vi "Run Command.vi"(8 "error in (no error)":errorcluster, 11 "Console Wrapper in":refnum<class "Console Wrapper.lvclass">) -> (0 "error out":errorcluster, 3 "Console Wrapper out":refnum<class "Console Wrapper.lvclass">)   [LabVIEW 2020, in "Console Wrapper.lvclass"]
doc: "Runs a built command in a specified working directory in the command line. It will wait until the command processing is finished and will not display the console window."
uses:
  Console Wrapper.lvclass
  Read Command.vi
  Read Working Directory.vi
  Write Standard Output.vi
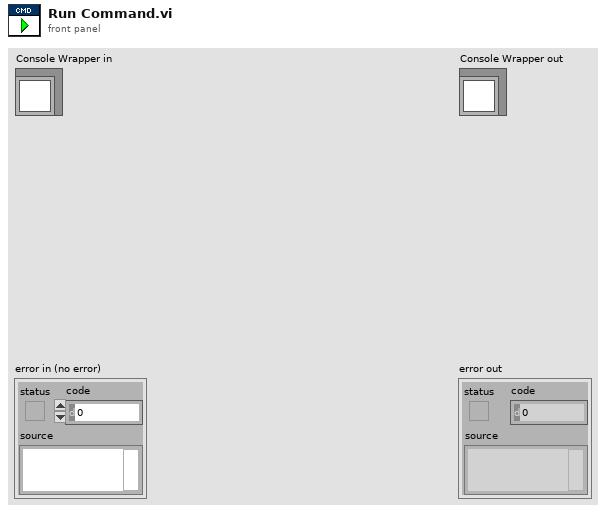
[diagram p1: front panel]
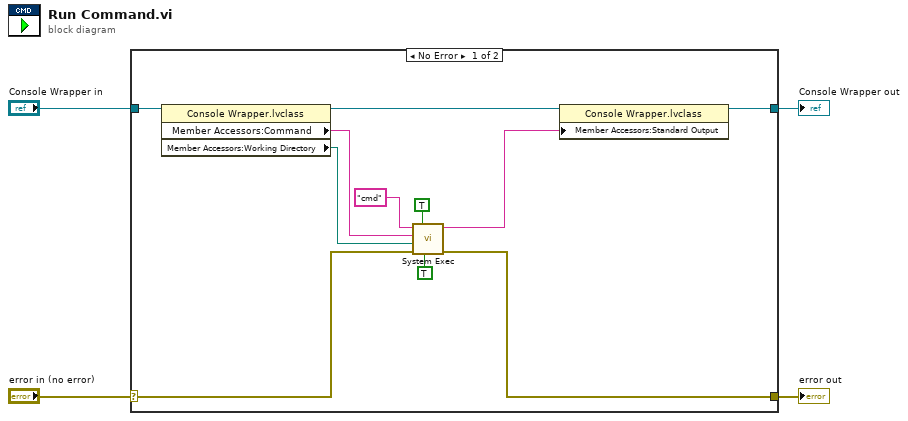
[diagram p0: block diagram]
diagram:
  n1 = case shown="No Error" "error in (no error)" {
    selector: "error in (no error)" -> [w6 w17]
    tunnel: [w5 w17] -> w3
    tunnel: [w13 w16] -> w1
    tunnel: "Console Wrapper in" -> [w15 w16]
    frame No Error {
      n2 = property class="Console Wrapper.lvclass"(reference=w15) -> (reference out=w14:refnum<class "Console Wrapper.lvclass">, "Member Accessors:Command"=w9:string, "Member Accessors:Working Directory"=w8:path)  [unwired: 1 in, 1 out]
      n3 = call <vilib>:"System Exec.vi"("run minimized? (F)"=TRUE, "wait until completion? (T)"=TRUE, "error in (no error)"=w6, "working directory"=w8, "standard input"=w9, "command line"="cmd") -> ("error out"=w5:errorcluster, "standard output"=w7:string)  [unwired: 2 in, 2 out]
      n4 = property class="Console Wrapper.lvclass"(reference=w14, "Member Accessors:Standard Output"=w7) -> (reference out=w13:refnum<class "Console Wrapper.lvclass">)  [unwired: 1 in, 1 out]
    }
    frame Error {
    }
  }
  "error out" <- w3
  "Console Wrapper out" <- w1
